vi "Insert Key Value Pair (Multi).vi"(7 "keys":string[](array[string]), 8 "error in (no error)":errorcluster, 10 "values":refnum<class "JSON Datatype.lvclass">[](array[class]), 11 "JSON Object in":refnum<class "JSON Object.lvclass">) -> (0 "error out":errorcluster, 3 "JSON Object out":refnum<class "JSON Object.lvclass">)   [LabVIEW 2015, in "LVJSON.lvlib" / "JSON Object.lvclass"]
uses:
  JSON Object.lvclass
  JSON Datatype/JSON Datatype.lvclass
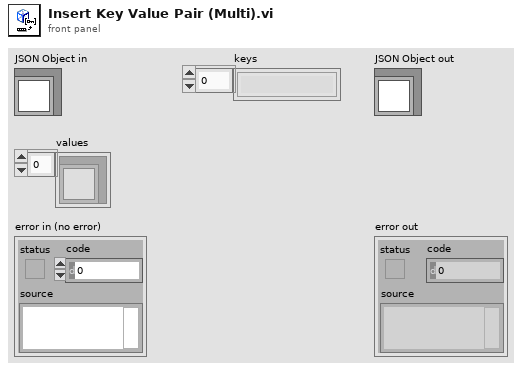
[diagram p1: front panel]
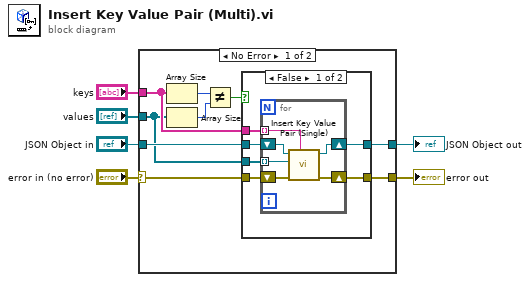
[diagram p0: block diagram]
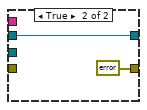
[diagram p2: hidden frame]
diagram:
  n1 = case shown="No Error" "error in (no error)" {
    selector: "error in (no error)" -> [w12 w31]
    tunnel: [w11 w31] -> w5
    tunnel: [w9 w30] -> w3
    tunnel: "JSON Object in" -> [w10 w30]
    tunnel: "keys" -> [w8 _]
    tunnel: "values" -> [w7 _]
    frame No Error {
      n2 = Array Size(array=w8) -> (size(s)=w15:i32)
      n3 = Array Size(array=w7) -> (size(s)=w14:i32)
      n4 = Not Equal?(x=w15, y=w14) -> (x != y?=w13:bool)
      n5 = case shown="False" w13 {
        tunnel: w12 -> [w19 _]
        tunnel: [w18 errorcluster {"status"=TRUE, "code"=-1000, "source"="There must be an equal number of keys and values"} ("error constant")] -> w11
        tunnel: w10 -> [w21 w28]
        tunnel: [w20 w28] -> w9
        tunnel: w8 -> [w17 _]
        tunnel: w7 -> [w16 _]
        frame False {
          n6 = for {
            shift-right: [w26] -> w20
            shift-left: w21 -> [w27]
            shift-right: [w24] -> w18
            shift-left: w19 -> [w25]
            tunnel: w17 -> [w23] mode=indexing
            tunnel: w16 -> [w22] mode=indexing
            n7 = call "Insert Key Value Pair (Single).vi"("key"=w23, "error in (no error)"=w25, "value"=w22, "JSON Object in"=w27) -> ("error out"=w24:errorcluster, "JSON Object out"=w26:refnum<class "JSON Object.lvclass">)  [unwired: 6 in]
          }
        }
        frame True {
        }
      }
    }
    frame Error {
    }
  }
  "error out" <- w5
  "JSON Object out" <- w3
